vi "Add_to_Comm_Var.vi"(9 "type":string, 10 "queue":variant, 11 "Type count":i32) -> ()   [LabVIEW 2010]
doc: "This VI implements the routine for adding the communication information of a new actor to the communication global variable. this information will be used by other actors to send messages between them.\n\nCreated by Davis Montenegro\nEPRI\n06-23-2017"
uses:
  Vars/Comm_Vars.vi
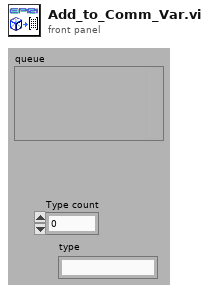
[diagram p1: front panel]
types:
  T1 = cluster{"actor_name":string, "actor_type":string, "queue":variant}[]
  T2 = cluster{"actor_name":string, "actor_type":string, "queue":variant}
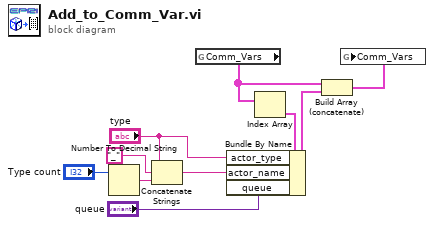
[diagram p0: block diagram]
diagram:
  n1 = Number To Decimal String(number="Type count") -> (decimal integer string=w8:string)  [unwired: 1 in]
  n2 = Concatenate Strings("type", "_", w8) -> (w6:string)
  n3 = global read "Comm_Vars.vi" "Comm_Vars"() -> (w5:T1)
  n4 = Index Array(array=w5) -> (element=w9:T2)  [unwired: 1 in]
  n5 = Bundle By Name(cluster=w9, "actor_type"="type", "actor_name"=w6, "queue"="queue") -> (w4:T2)
  n6 = Build Array (concatenate)(w5, w4) -> (w3:T1)
  n7 = global write "Comm_Vars.vi" "Comm_Vars"(w3) -> ()
